vi "Results_FromPositionMove.vi"(11 "Results":dbl[](array[numeric])) -> (0 "Steps_Generated":dbl, 1 "Velocity":dbl, 2 "Position":dbl, 3 "Axis_Number":dbl)   [LabVIEW 2017, in "WordManipulationLibrary.lvlib"]
uses:
  WordManipulationLibrary.lvlib
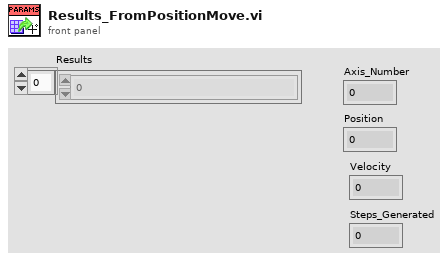
[diagram p1: front panel]
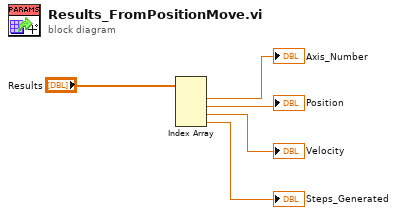
[diagram p0: block diagram]
diagram:
  n1 = Index Array(array="Results") -> (element #1=→"Axis_Number":dbl, element #2=→"Position":dbl, element #3=→"Velocity":dbl, element #4=→"Steps_Generated":dbl)  [unwired: 4 in]
